vi "Do That Thang.vi"(8 "error in (no error)":errorcluster, 9 "Lookup Table":refnum<data-value>, 11 "iTest Step in":refnum<class "iTest Step.lvclass">) -> (0 "error out":errorcluster, 3 "iTest Step out":refnum<class "iTest Step.lvclass">)   [LabVIEW 2020, in "Test Executive.lvlib" / "Parallelizer Example.lvlib" / "iTest Step.lvclass"]
uses:
  <vilib>/gpm_packages/@cs/test-executive/Source/Sandbox/Parallelizer Example/iTest Step/iTest Step.lvclass
  <vilib>/gpm_packages/@cs/lookup-table/Source/LookupTable/LookupTable.lvclass
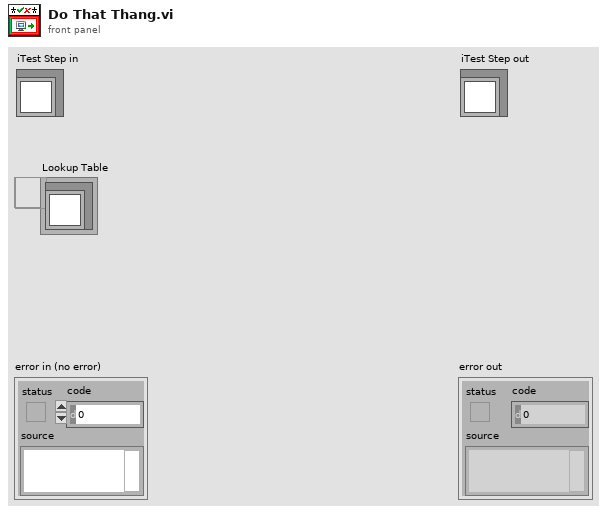
[diagram p1: front panel]
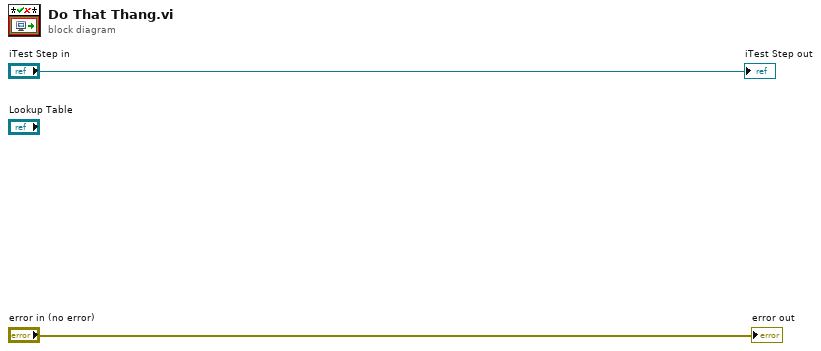
[diagram p0: block diagram]
diagram:
  "error out" <- "error in (no error)"
  "iTest Step out" <- "iTest Step in"
